vi "Axis_Offset.vi"(3 "Position In":sgl[](array[numeric])=[0.0, 0.0, 0.0] format="%#.2f", 4 "Axis":T1, 5 "Roll-Pitch-Yaw":sgl[](array[numeric]) caption="Model       Roll         Pitch        Yaw (deg)" format="%#.2f", 6 "Traverse Name":string) -> (0 "Correct array":bool, 1 "Offset":sgl, 2 "Offset Array":sgl[](array[numeric]))   [LabVIEW 2015]
uses:
  Route mapping/Axis.ctl
  Globals/Constants_global.vi
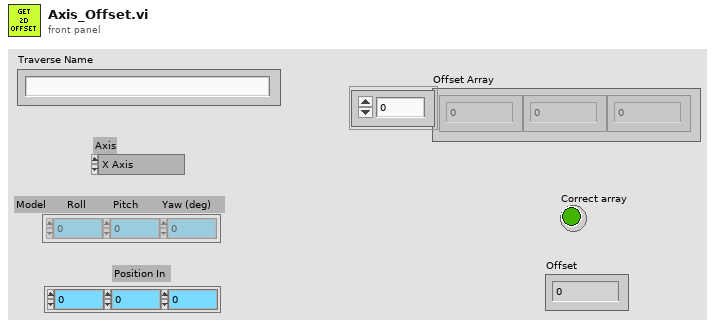
[diagram p1: front panel]
types:
  T1 = typedef "Axis.ctl" = enum16{"X Axis", "X Axis -ve", "Y Axis", "Y Axis -ve", "Z Axis", "Z Axis -ve"}
  T2 = enum16{"To Traverse Coordinates", "To User Coordinates"}
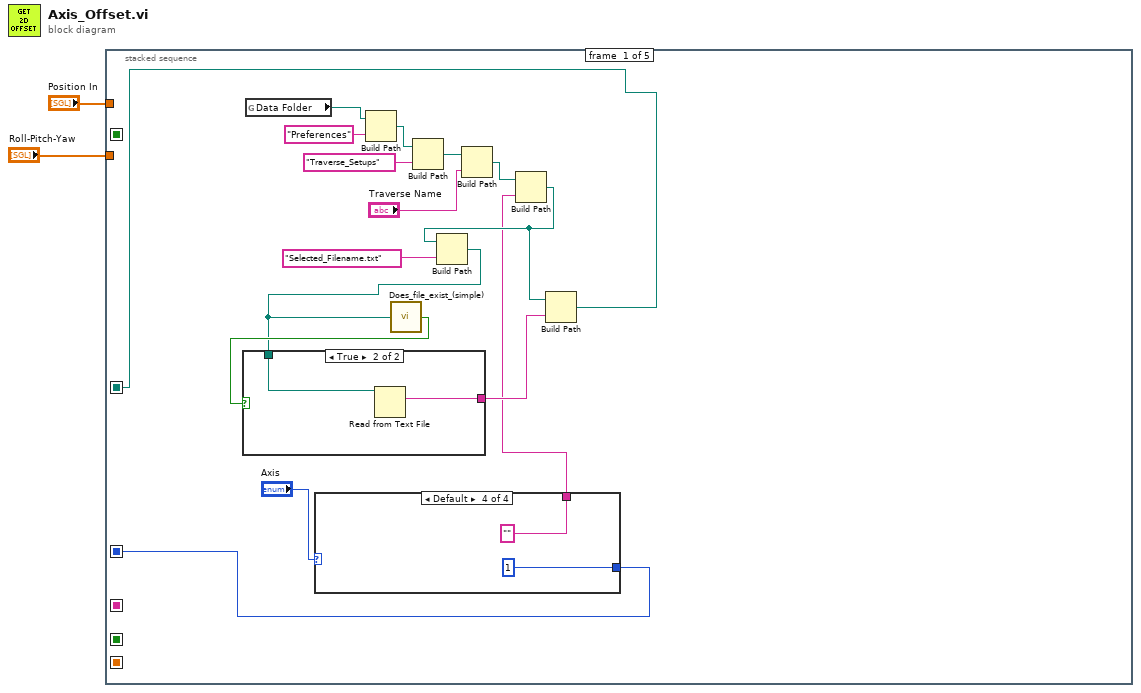
[diagram p0: block diagram]
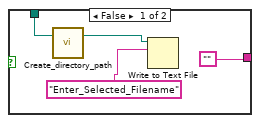
[diagram p2: hidden frame]
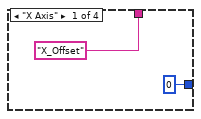
[diagram p3: hidden frame]
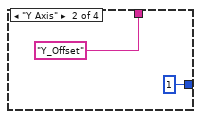
[diagram p4: hidden frame]
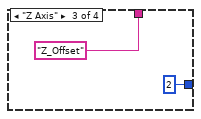
[diagram p5: hidden frame]
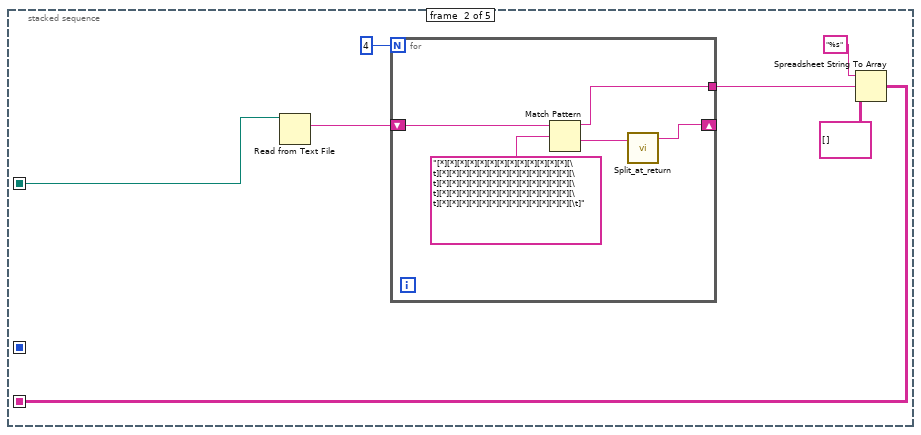
[diagram p6: hidden frame]
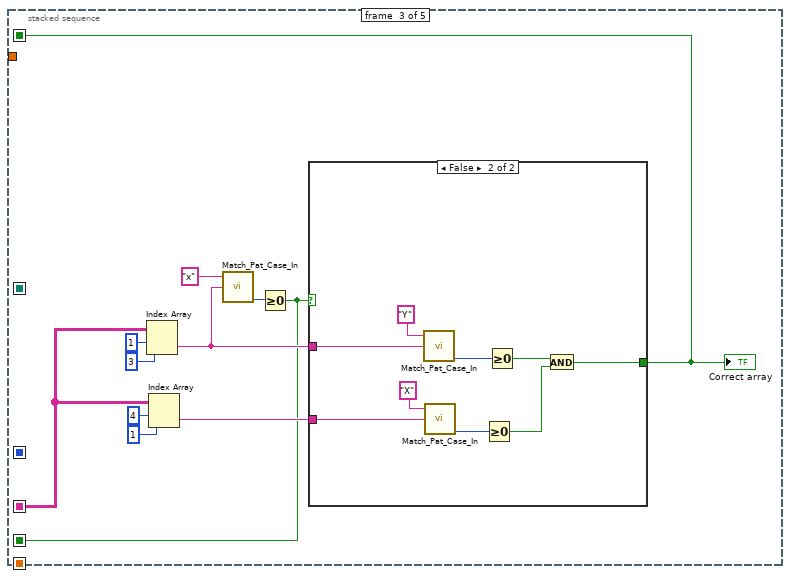
[diagram p7: hidden frame]
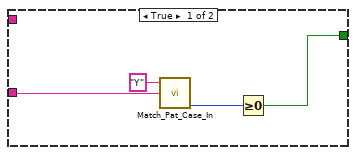
[diagram p8: hidden frame]
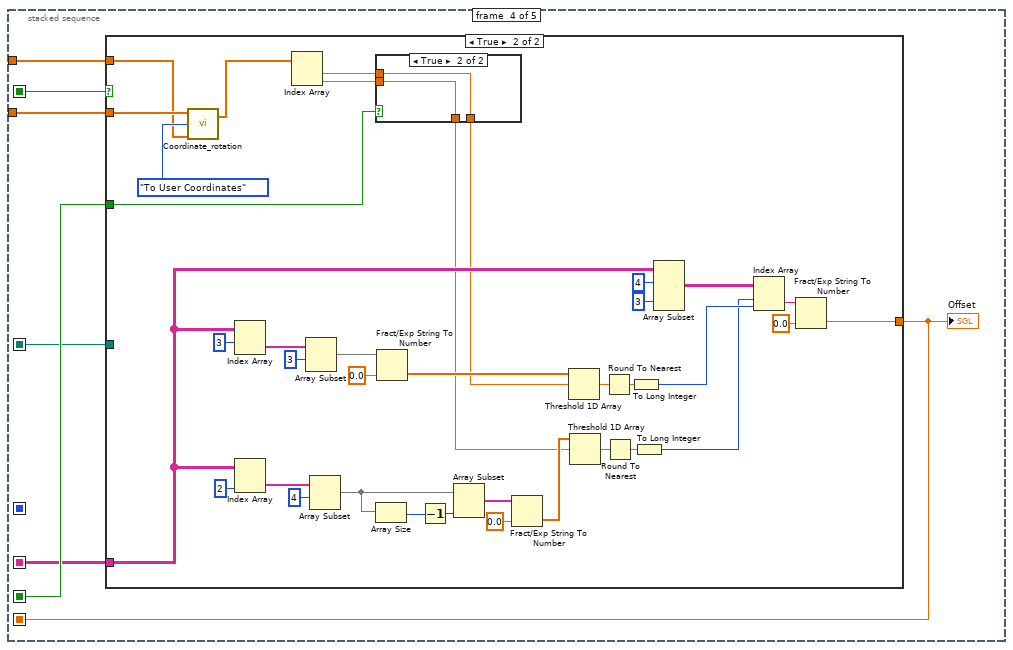
[diagram p9: hidden frame]
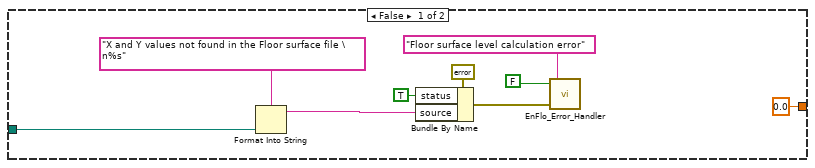
[diagram p10: hidden frame]
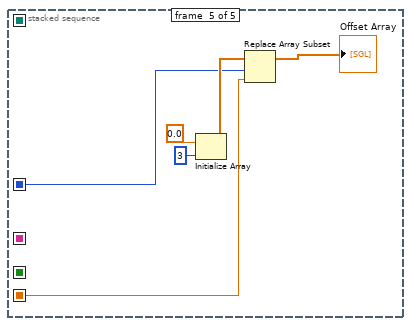
[diagram p12: hidden frame]
diagram:
  n1 = stacked-sequence {
    seq-local: [_ w34 _ _ _] -> [_ _ w50 w70 _]
    seq-local: [_ _ w46 _ _] -> [_ _ _ w75 _]
    seq-local: [_ _ _ w72 _] -> [_ _ _ _ w126]
    seq-local: [_ _ w45 _ _] -> [_ _ _ w73 _]
    seq-local: [w4 _ _ _ _] -> [_ w33 _ w71 _]
    seq-local: [w3 _ _ _ _] -> [_ _ _ _ w128]
    tunnel: "Position In" -> [_ _ _ w74 _]
    tunnel: "Roll-Pitch-Yaw" -> [_ _ _ w69 _]
    frame #0 {
      n2 = global read "Constants_global.vi" "Data Folder"() -> (w6:path)
      n3 = case shown="Default" "Axis" {
        tunnel: ["X_Offset" ("name or relative path") "Y_Offset" ("name or relative path") "Z_Offset" ("name or relative path") "" ("name or relative path")] -> w14
        tunnel: [0 ("index") 1 ("index") 2 ("index") 1 ("index")] -> w3
        frame "X Axis" {
        }
        frame "Y Axis" {
        }
        frame "Z Axis" {
        }
        frame Default {
        }
      }
      n4 = Build Path(base path=w6, name or relative path="Preferences") -> (appended path=w8:path)
      n5 = Build Path(base path=w8, name or relative path="Traverse_Setups") -> (appended path=w9:path)
      n6 = Build Path(base path=w9, name or relative path="Traverse Name") -> (appended path=w13:path)
      n7 = Build Path(base path=w13, name or relative path=w14) -> (appended path=w15:path)
      n8 = Build Path(base path=w15, name or relative path="Selected_Filename.txt" ("Substring")) -> (appended path=w16:path)
      n9 = call "Does_file_exist_(simple).vi"("Pathname"=w16) -> ("exists?"=w17:bool)
      n10 = case shown="True" w17 {
        tunnel: w16 -> [w21 w24]
        tunnel: ["" w23] -> w18
        frame False {
          n11 = call "Create_directory_path.vi"("Path name"=w21) -> ("Path name Out"=w20:path)  [unwired: 1 in, 1 out]
          n12 = Write to Text File(file (use dialog)=w20, text="Enter_Selected_Filename" ("Substring")) -> ()  [unwired: 2 in, 3 out]
        }
        frame True {
          n13 = Read from Text File(file (use dialog)=w24) -> (text=w23:string)  [unwired: 3 in, 3 out]
        }
      }
      n14 = Build Path(base path=w15, name or relative path=w18) -> (appended path=w4:path)
    }
    frame #1 {
      n15 = Read from Text File(file (use dialog)=w33) -> (text=w39:string)  [unwired: 3 in, 3 out]
      n16 = for {
        N: 4 -> [_]
        shift-right: [w41] -> _
        shift-left: w39 -> [w42]
        tunnel: [w40] -> w36
        n17 = Match Pattern(string=w42, regular expression="[*][*][*][*][*][*][*][*][*][*][*][*][*][\t][*][*][*][*][*][*][*][*][*][*][*][*][*][\t][*][*][*][*][*][*][*][*][*][*][*][*][*][\t][*][*][*][*][*][*][*][*][*][*][*][*][*][\t][*][*][*][*][*][*][*][*][*][*][*][*][*][\t]" ("String")) -> (before substring=w40:string, after substring=w43:string)  [unwired: 3 out]
        n18 = call "Split_at_return.vi"("String"=w43) -> ("after substring"=w41:string)  [unwired: 1 in, 3 out]
      }
      n19 = Spreadsheet String To Array(format string="%s", spreadsheet string=w36, array type (2D Dbl)=string[][] []) -> (array=w34:string[][])  [unwired: 1 in]
    }
    frame #2 {
      n20 = Index Array(array=w50, index (row)=1, index (col)=3) -> (element=w48:string)
      n21 = Index Array(array=w50, index (row)=4, index (col)=1) -> (element=w49:string)
      n22 = call "Match_Pat_Case_In.vi"("String to match"="x", "String"=w48) -> ("offset past match"=w47:i32)  [unwired: 1 in, 3 out]
      n23 = Greater Or Equal To 0?(x=w47) -> (x >= 0?=w46:bool)
      n24 = case shown="False" w46 {
        tunnel: w49 -> [w58 w67]
        tunnel: w48 -> [_ w65]
        tunnel: [w56 w60] -> w45
        frame True {
          n25 = call "Match_Pat_Case_In.vi"("String to match"="Y", "String"=w58) -> ("offset past match"=w57:i32)  [unwired: 1 in, 3 out]
          n26 = Greater Or Equal To 0?(x=w57) -> (x >= 0?=w56:bool)
        }
        frame False {
          n27 = call "Match_Pat_Case_In.vi"("String to match"="Y", "String"=w65) -> ("offset past match"=w64:i32)  [unwired: 1 in, 3 out]
          n28 = call "Match_Pat_Case_In.vi"("String to match"="X", "String"=w67) -> ("offset past match"=w63:i32)  [unwired: 1 in, 3 out]
          n29 = Greater Or Equal To 0?(x=w63) -> (x >= 0?=w62:bool)
          n30 = Greater Or Equal To 0?(x=w64) -> (x >= 0?=w61:bool)
          n31 = And(x=w61, y=w62) -> (x .and. y?=w60:bool)
        }
      }
      "Correct array" <- w45
    }
    frame #3 {
      n32 = case shown="True" w73 {
        tunnel: w70 -> [_ w107]
        tunnel: w75 -> [_ w106]
        tunnel: [sgl 0.0 w101] -> w72
        tunnel: w74 -> [_ w86]
        tunnel: w71 -> [w78 _]
        tunnel: w69 -> [_ w87]
        frame False {
          n33 = Format Into String(format string="X and Y values not found in the Floor surface file \n%s", w78) -> (resulting string=w76:string)  [unwired: 2 in, 1 out]
          n34 = Bundle By Name(cluster=errorcluster {"status"=FALSE, "code"=0, "source"=""} ("error in (no error)"), "status"=TRUE, "source"=w76) -> (w81:errorcluster)
          n35 = call "EnFlo_Error_Handler.vi"("error in (no error)"=w81, "Error Type"="Floor surface level calculation error", "Dialog Box (T)"=FALSE) -> ()  [unwired: 3 out]
        }
        frame True {
          n36 = call "Coordinate_rotation.vi"("Roll-Pitch-Yaw"=w87, "Input Position"=w86, "Mode"=T2."To User Coordinates") -> ("Output Position"=w85:sgl[])  [unwired: 2 in, 1 out]
          n37 = Index Array(array=w107, index (row)=3) -> (element=w120:string[])  [unwired: 1 in]
          n38 = Index Array(array=w107, index (col)=2 ("index (row)")) -> (element=w116:string[])  [unwired: 1 in]
          n39 = Index Array(array=w85) -> (element #1=w103:sgl, element #2=w102:sgl)  [unwired: 2 in]
          n40 = Array Subset(array=w120, index=3) -> (w113:string[])  [unwired: 1 in]
          n41 = Array Subset(array=w116, index=4) -> (w93:string[])  [unwired: 1 in]
          n42 = case shown="True" w106 {
            tunnel: w103 -> [w123 w125]
            tunnel: [w122 w125] -> w105
            tunnel: [w123 w124] -> w104
            tunnel: w102 -> [w122 w124]
            frame False {
            }
            frame True {
            }
          }
          n43 = Array Size(array=w93) -> (size(s)=w95:i32)
          n44 = Fract/Exp String To Number(string=w113, default (0 dbl)=sgl 0.0 ("default (0 DBL)")) -> (number=w112:sgl[])  [unwired: 2 in, 1 out]
          n45 = Decrement(x=w95) -> (x-1=w94:i32)
          n46 = Array Subset(array=w93, length=w94) -> (w92:string[])  [unwired: 1 in]
          n47 = Fract/Exp String To Number(string=w92, default (0 dbl)=sgl 0.0 ("default (0 DBL)")) -> (number=w109:sgl[])  [unwired: 2 in, 1 out]
          n48 = Threshold 1D Array(2:w105, 3:w112) -> (0:w111:sgl)  [unwired: 1 in]
          n49 = Threshold 1D Array(2:w104, 3:w109) -> (0:w110:sgl)  [unwired: 1 in]
          n50 = Round To Nearest(number=w111) -> (nearest integer value=w100:sgl)
          n51 = Round To Nearest(number=w110) -> (nearest integer value=w99:sgl)
          n52 = To Long Integer(number=w100) -> (32bit integer=w97:i32)
          n53 = To Long Integer(number=w99) -> (32bit integer=w96:i32)
          n54 = Array Subset(array=w107, index (row)=4 ("index"), index (col)=3 ("index")) -> (w98:string[][])  [unwired: 2 in]
          n55 = Index Array(array=w98, index (row)=w96, index (col)=w97) -> (element=w108:string)
          n56 = Fract/Exp String To Number(string=w108, default (0 dbl)=sgl 0.0 ("default (0 DBL)")) -> (number=w101:sgl)  [unwired: 2 in, 1 out]
        }
      }
      "Offset" <- w72
    }
    frame #4 {
      n57 = Initialize Array(sgl 0.0, 3 ("dimension size")) -> (w129:sgl[])
      n58 = Replace Array Subset(array=w129, new element=w126, index=w128) -> (→"Offset Array":sgl[])
    }
  }
